vi "Get Single.vi"(8 "error in":errorcluster, 10 "CMD":string="R1") -> (0 "error out":errorcluster, 2 "DataOut":sgl)   [LabVIEW 2015, in "Text Device Session.lvclass"]
doc: "Write to serial port and retrieve a floating point number."
uses:
  Text Communication/Text Device Session.lvclass
  <userlib>/_Session Fwk/Typedefs/Session Handle.ctl
  <userlib>/_Session Fwk/Session - Root.lvclass
panel:
  out "handle out":T1
  in  "handle in":T1
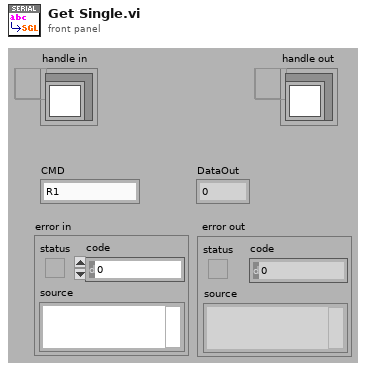
[diagram p1: front panel]
types:
  T1 = typedef "Session - Root.lvclass/Session Handle.ctl" = refnum<data-value>
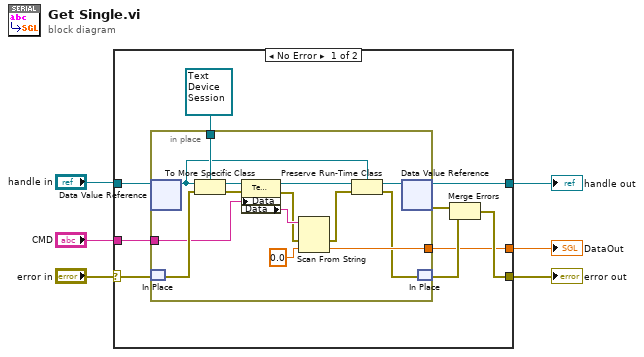
[diagram p0: block diagram]
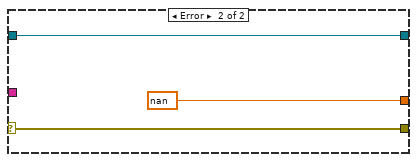
[diagram p2: hidden frame]
diagram:
  n1 = case shown="No Error" "error in" {
    selector: "error in" -> [w10 w31]
    tunnel: "handle in" -> [w15 w32]
    tunnel: [w14 w32] -> w4
    tunnel: [w11 w31] -> w1
    tunnel: "CMD" -> [w9 _]
    tunnel: [w8 sgl nan ("default value 1")] -> w3
    frame No Error {
      n2 = in-place {
        in-place-border: w9 -> [w23]
        in-place-border: [w28] -> w8
        in-place-border: refnum<class "Text Device Session.lvclass"> refnum ("Text Session") -> [w26]
        n3 = in-place-dvr #1(w15) -> (w19:refnum<class "Session - Root.lvclass">)  [unwired: 1 out]
        n4 = in-place-match #2(w10) -> (w27:errorcluster)
        n5 = To More Specific Class(target class=w26, reference=w19, error in=w27) -> (specific class reference=w25:refnum<class "Text Device Session.lvclass">, error out=w24:errorcluster)
        n6 = property class="Text Session"(reference=w25, error in=w24, "Data"=w23) -> (reference out=w20:refnum<class "Text Device Session.lvclass">, error out=w21:errorcluster, "Data"=w22:string)
        n7 = Scan From String(input string=w22, error in=w21, default 1=sgl 0.0 ("default value 1")) -> (error out=w17:errorcluster, output 1=w28:sgl)  [unwired: 2 in, 2 out]
        n8 = Preserve Run-Time Class(object in=w20, error in=w17, 2:w19) -> (object out=w18:refnum<class "Session - Root.lvclass">, error out=w16:errorcluster)
        n9 = in-place-dvr #1(w18) -> (w14:T1, w12:errorcluster)
        n10 = in-place-match #2(w16) -> (w13:errorcluster)
      }
      n11 = Merge Errors(w12, w13) -> (w11:errorcluster)
    }
    frame Error {
    }
  }
  "error out" <- w1
  "DataOut" <- w3
  "handle out" <- w4
